vi "Save Data (Incomplete Collection).vi"(7 "File Name":string, 8 "error in (no error)":errorcluster, 9 "Audio":dynamicdata(waveform), 10 "Save Data":dynamicdata(waveform), 11 "Pulse":dbl) -> (0 "error out":errorcluster, 3 "cancelled":bool)   [LabVIEW 2018, in "CollectionSupport.lvlib"]
uses:
  CollectionSupport.lvlib
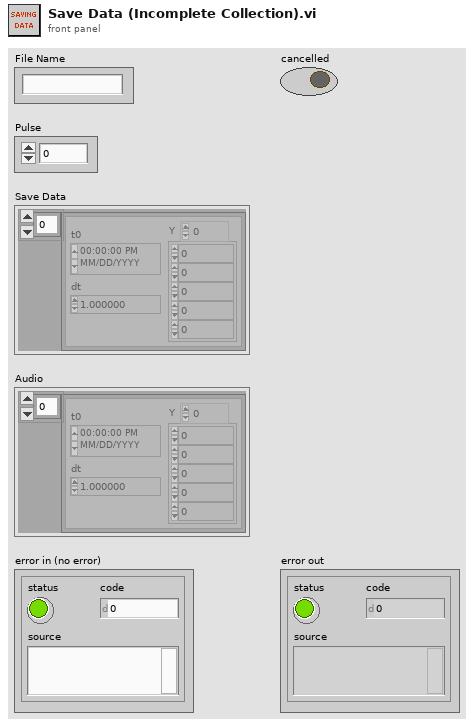
[diagram p1: front panel]
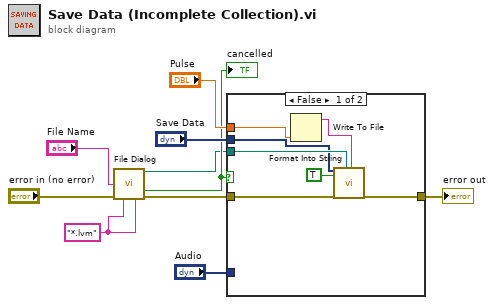
[diagram p0: block diagram]
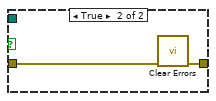
[diagram p2: hidden frame]
diagram:
  w7 = "*.lvm" ("pattern (all files)")
  n1 = call "File Dialog"("default name"="File Name", "error in"="error in (no error)", "pattern (all files)"=w7, "pattern label"=w7) -> ("selected path"=w4:path, "cancelled"=w5:bool, "error out"=w3:errorcluster)  [unwired: 8 in, 1 out]
  "cancelled" <- w5
  n2 = case shown="False" w5 {
    tunnel: [w11 w18] -> w1
    tunnel: w3 -> [w17 w19]
    tunnel: w4 -> [w15 _]
    tunnel: "Audio" -> [_ _]
    tunnel: "Pulse" -> [w13 _]
    tunnel: "Save Data" -> [w12 _]
    frame False {
      n3 = Format Into String(w13) -> (resulting string=w14:string)  [unwired: 3 in, 1 out]
      n4 = call "Write To File"("Signals"=w12, "Reset"=TRUE, "error in (no error)"=w17, "Filename"=w15, "Comment"=w14) -> ("error out"=w11:errorcluster)  [unwired: 12 in, 2 out]
    }
    frame True {
      n5 = call <vilib>:"Clear Errors.vi"("error in (no error)"=w19) -> ("error out"=w18:errorcluster)  [unwired: 5 in, 1 out]
    }
  }
  "error out" <- w1
